vi "BeamDiagnosticFGV.vi"(10 "BeamDiagnosticCamControl":enum16{"Set", "Get"}(ring), 11 "setCamStop":bool) -> (3 "getCamStop":bool)   [LabVIEW 2010]
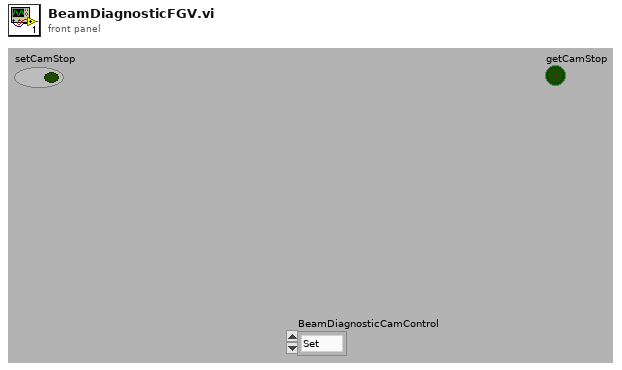
[diagram p1: front panel]
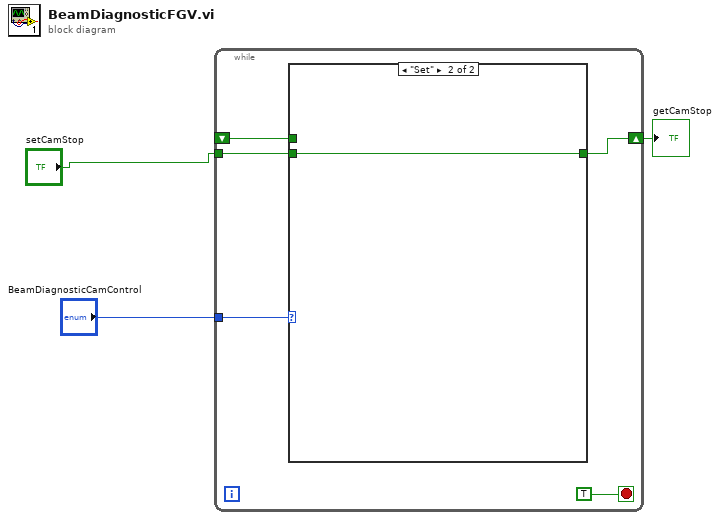
[diagram p0: block diagram]
diagram:
  n1 = while {
    tunnel: "BeamDiagnosticCamControl" -> [w8]
    tunnel: "setCamStop" -> [w7]
    shift-right: [w6] -> w1
    shift-left: _ -> [w5]
    stop <- TRUE stop-if-true
    n2 = case shown="\"Set\"" w8 {
      tunnel: w7 -> [_ w10]
      tunnel: [w9 w10] -> w6
      tunnel: w5 -> [w9 _]
      frame "Get" {
      }
      frame "Set" {
      }
    }
  }
  "getCamStop" <- w1
